vi "Mixed Mode Parameters Popup.vi"(11 "error in (no error)":errorcluster) -> (4 "L1 Param":bool, 6 "L1 Stiff":bool, 8 "L2 Param":bool, 10 "L2 Stiff":bool, 15 "error out":errorcluster)   [LabVIEW 2013]
uses:
  lib/Data Access Objects/Metadata/Cartesian Point.ctl
  lib/Data Access Objects/Metadata/Cartesian Force Vector.ctl
  lib/Data Access Objects/Metadata/Cartesian Force Matrix.ctl
  lib/Data Access Objects/Metadata/Persistant DAO Actions.ctl
  lib/Data Access Objects/Metadata/LBCB Number.ctl
panel:
  in  "Tab Control":enum32{"Parameters", "Stiffness"}(tab)
  in  "Max Increment L1":T1 caption="Max Increment"
  in  "Jacobian Gain L1":T1 caption="Jacobian Gain"
  in  "Force Error Range L1":T2 caption="Force Error Range"
  in  "Max Increment L2":T1 caption="Max Increment"
  in  "Jacobian Gain L2":T1 caption="Jacobian Gain"
  in  "Force Error Range L2":T2 caption="Force Error Range"
  in  "Limit L2 Label 2":string="LBCB 2"
  in  "Jacobian Diagonal LBCB2":dbl[](array[numeric])
  in  "Jacobian Diagonal LBCB1":dbl[](array[numeric])
  in  "Stiffness Limit LBCB2":T3
  in  "Stiffness Limit LBCB1":T3
  in  "Ok":bool
  # "LBCB 1"
  # "dDx"
  # "dDx"
  # "dDy"
  # "dDy"
  # "dDz"
  # "dDz"
  # "dRx"
  # "dRx"
  # "dRy"
  # "dRy"
  # "dRz"
  # "dRz"
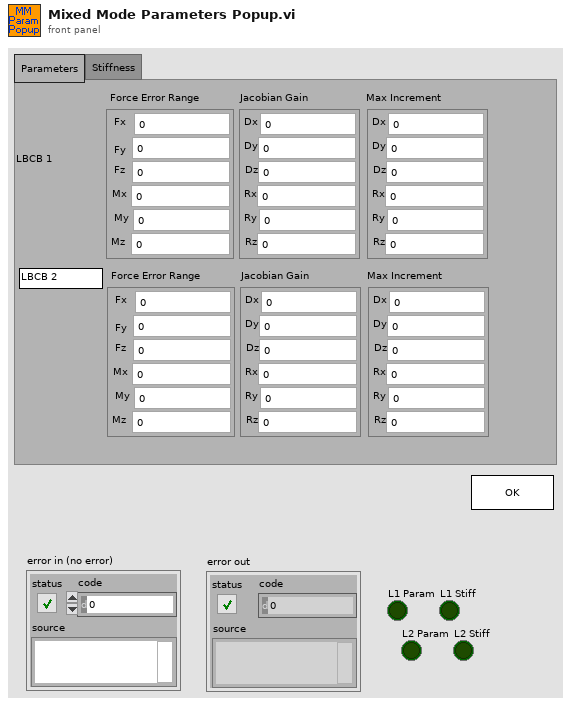
[diagram p1: front panel]
types:
  T1 = typedef "Cartesian Point.ctl" = cluster{"Dx":dbl, "Dy":dbl, "Dz":dbl, "Rx":dbl, "Ry":dbl, "Rz":dbl}
  T2 = typedef "Cartesian Force Vector.ctl" = cluster{"Fx":dbl, "Fy":dbl, "Fz":dbl, "Mx":dbl, "My":dbl, "Mz":dbl}
  T3 = typedef "Cartesian Force Matrix.ctl" = cluster{"Lower":T2, "Upper":T2}
  T4 = typedef "LBCB Number.ctl" = enum16{"LBCB1", "LBCB2"}
  T5 = typedef "Persistant DAO Actions.ctl" = enum16{"Init", "Get", "Set", "Load", "Save"}
  T6 = typedef "Stiffness Matrix.ctl" = dbl[][]
  T7 = typedef "Cartesian Matrix.ctl" = cluster{"Lower":T1, "Upper":T1}
  T8 = typedef "Number Of LBCBs.ctl" = enum16{"1", "2"}
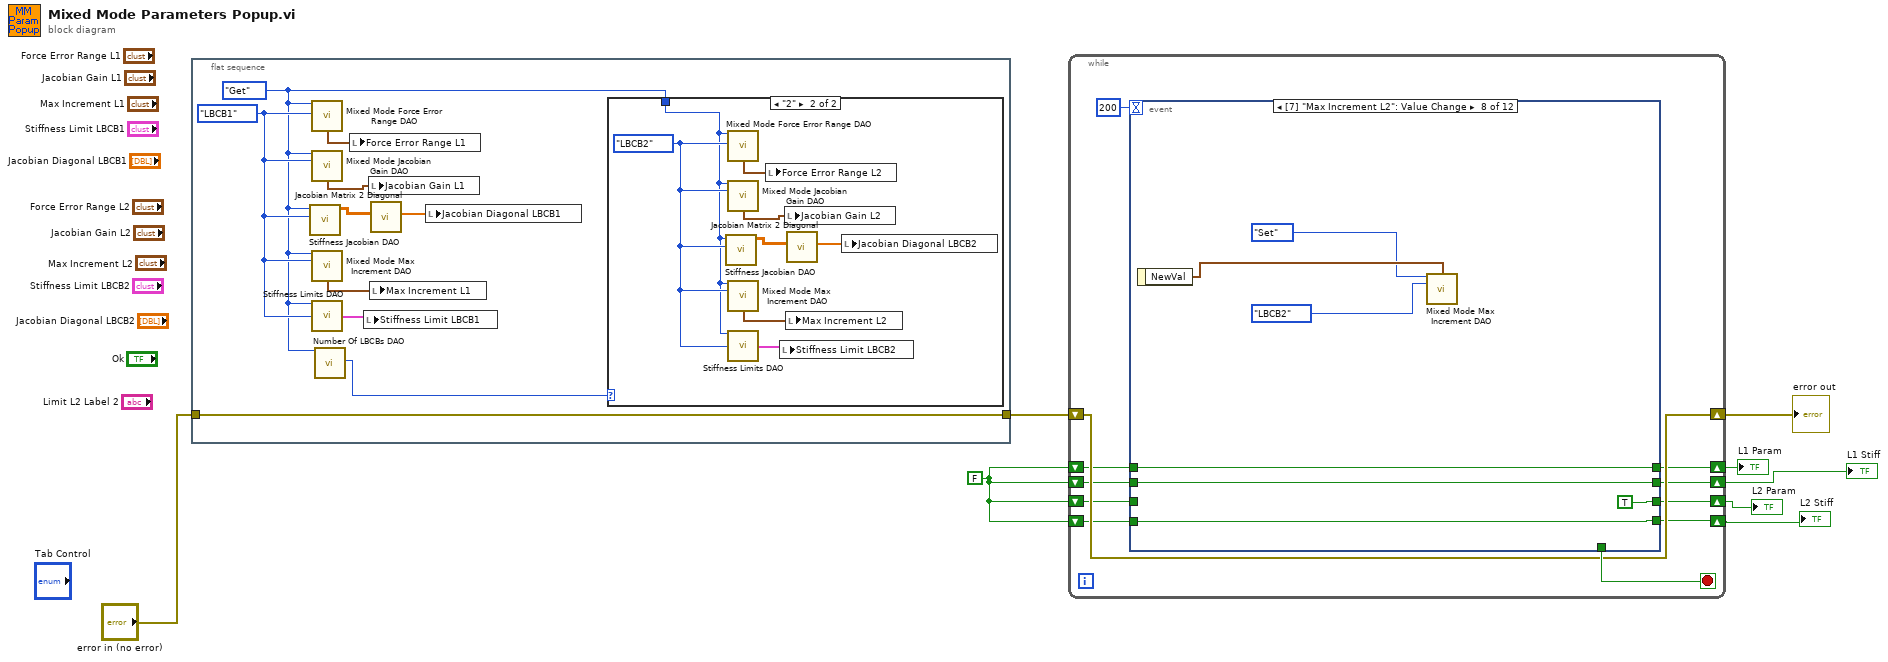
[diagram p0: block diagram]
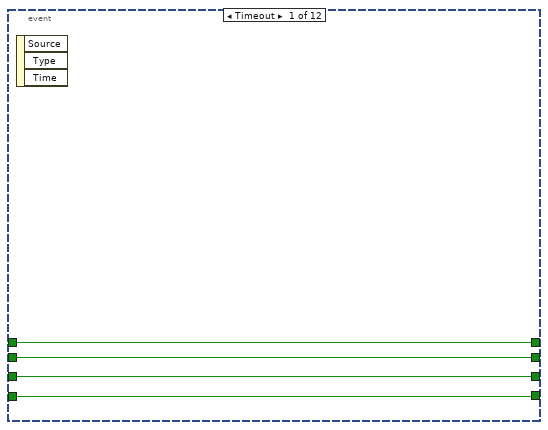
[diagram p2: hidden frame]
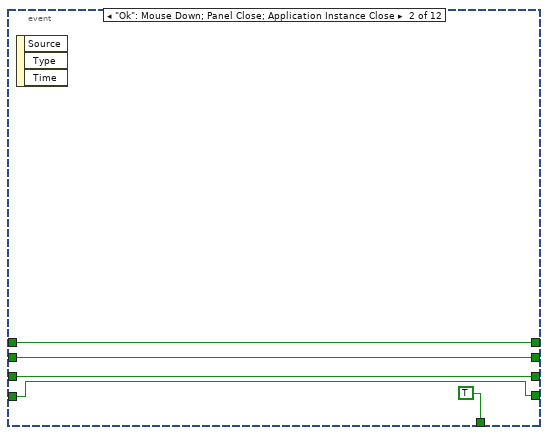
[diagram p3: hidden frame]
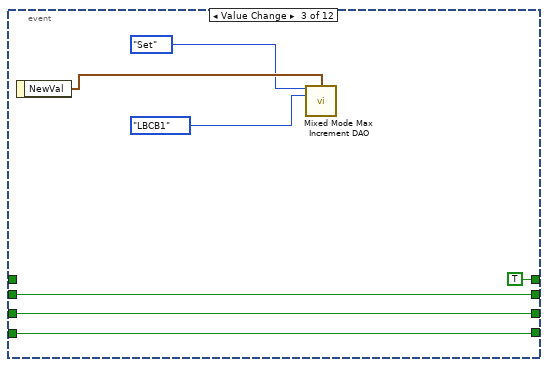
[diagram p4: hidden frame]
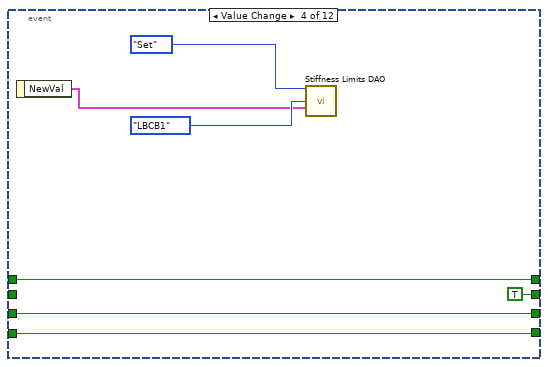
[diagram p5: hidden frame]
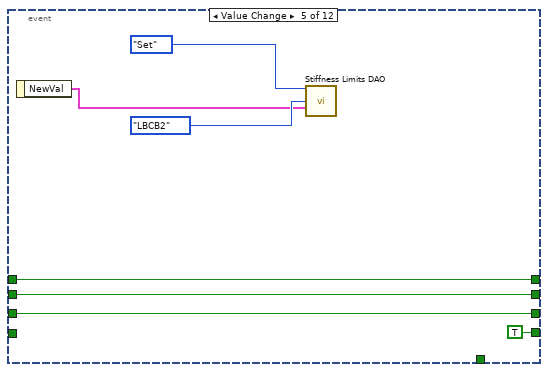
[diagram p6: hidden frame]
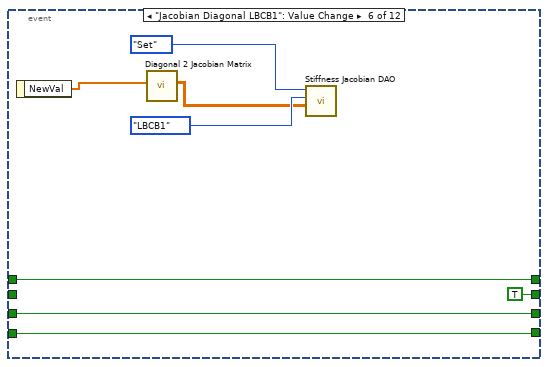
[diagram p7: hidden frame]
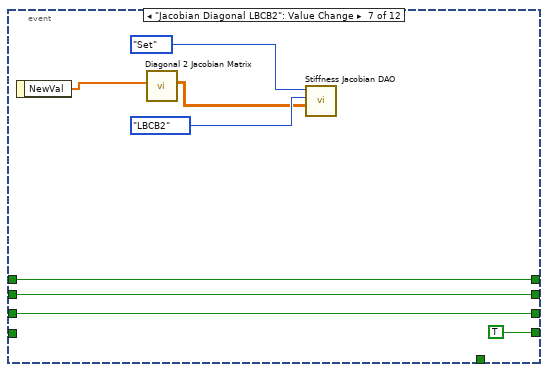
[diagram p8: hidden frame]
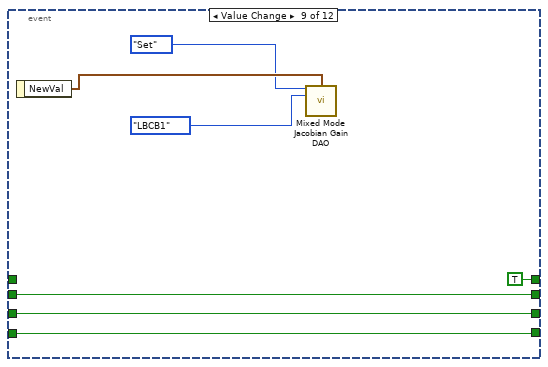
[diagram p9: hidden frame]
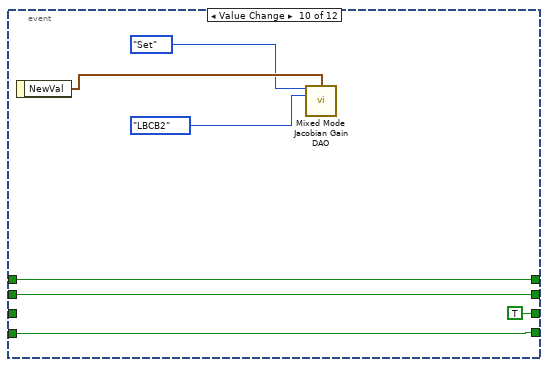
[diagram p10: hidden frame]
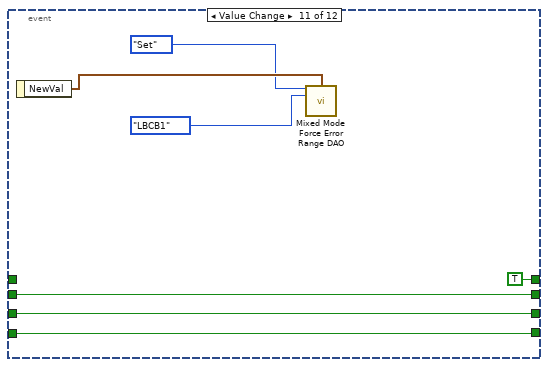
[diagram p11: hidden frame]
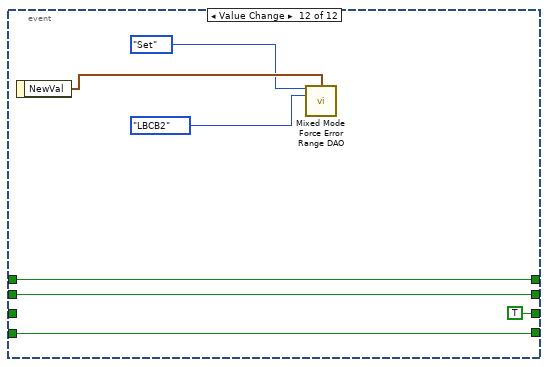
[diagram p12: hidden frame]
diagram:
  w5 = FALSE
  n1 = flat-sequence {
    tunnel: "error in (no error)" -> [w9]
    tunnel: [w9] -> w7
    frame #0 {
      w12 = LBCB_Number."LBCB1" ("LBCB Number")
      w10 = Persistant_DAO_Actions."Get" ("Force Error Range Actions")
      n2 = call "Stiffness Jacobian DAO.vi"("LBCB Number"=w12, "Actions"=w10) -> ("Stiffness Jacobian Out"=w16:T6)  [unwired: 3 in, 6 out]
      n3 = call "Mixed Mode Force Error Range DAO.vi"("Force Error Range Actions"=w10, "LBCB Number"=w12) -> ("Force Error Range Out"=w18:T1)  [unwired: 3 in, 10 out]
      n4 = call "Mixed Mode Jacobian Gain DAO.vi"("Jacobian Gain Actions"=w10, "LBCB Number"=w12) -> ("Jacobian Gain Out"=w17:T1)  [unwired: 3 in, 10 out]
      n5 = call "Mixed Mode Max Increment DAO.vi"("Max Increment Actions"=w10, "LBCB Number"=w12) -> ("Max Increment Out"=w14:T1)  [unwired: 3 in, 10 out]
      n6 = call "Stiffness Limits DAO.vi"("Actions"=w10, "ID"=w12) -> ("Stiffness Limit Out"=w13:T7)  [unwired: 11 in, 2 out]
      n7 = call "Number Of LBCBs DAO.vi"("Actions"=w10) -> ("Number of\nLBCBs Out"=w11:T8)  [unwired: 13 in, 5 out]
      n8 = local write "Force Error Range L1"(w18) -> ()
      n9 = local write "Stiffness Limit LBCB1"(w13) -> ()
      n10 = local write "Jacobian Gain L1"(w17) -> ()
      n11 = local write "Max Increment L1"(w14) -> ()
      n12 = call "Jacobian Matrix 2 Diagonal.vi"("Stiffness Jacobian In"=w16) -> ("Jacobian Diagonal Out"=w15:dbl[])  [unwired: 10 in]
      n13 = local write "Jacobian Diagonal LBCB1"(w15) -> ()
      n14 = case shown="\"2\"" w11 {
        tunnel: w10 -> [_ w19]
        frame "1", Default {
        }
        frame "2" {
          w26 = LBCB_Number."LBCB2" ("LBCB Number")
          n15 = call "Stiffness Jacobian DAO.vi"("LBCB Number"=w26, "Actions"=w19) -> ("Stiffness Jacobian Out"=w22:T6)  [unwired: 3 in, 6 out]
          n16 = call "Mixed Mode Force Error Range DAO.vi"("Force Error Range Actions"=w19, "LBCB Number"=w26) -> ("Force Error Range Out"=w20:T1)  [unwired: 3 in, 10 out]
          n17 = call "Mixed Mode Jacobian Gain DAO.vi"("Jacobian Gain Actions"=w19, "LBCB Number"=w26) -> ("Jacobian Gain Out"=w21:T1)  [unwired: 3 in, 10 out]
          n18 = call "Mixed Mode Max Increment DAO.vi"("Max Increment Actions"=w19, "LBCB Number"=w26) -> ("Max Increment Out"=w24:T1)  [unwired: 3 in, 10 out]
          n19 = call "Stiffness Limits DAO.vi"("Actions"=w19, "ID"=w26) -> ("Stiffness Limit Out"=w25:T7)  [unwired: 11 in, 2 out]
          n20 = local write "Force Error Range L2"(w20) -> ()
          n21 = local write "Stiffness Limit LBCB2"(w25) -> ()
          n22 = local write "Jacobian Gain L2"(w21) -> ()
          n23 = local write "Max Increment L2"(w24) -> ()
          n24 = call "Jacobian Matrix 2 Diagonal.vi"("Stiffness Jacobian In"=w22) -> ("Jacobian Diagonal Out"=w23:dbl[])  [unwired: 10 in]
          n25 = local write "Jacobian Diagonal LBCB2"(w23) -> ()
        }
      }
    }
  }
  n26 = while {
    shift-right: [w35] -> w6
    shift-left: w7 -> [w35]
    shift-right: [w27] -> w4
    shift-left: w5 -> [w30]
    shift-right: [w28] -> w3
    shift-left: w5 -> [w31]
    shift-right: [w29] -> w2
    shift-left: w5 -> [w33]
    shift-right: [w34] -> w1
    shift-left: w5 -> [w32]
    stop <- w36 stop-if-true
    n27 = event shown="[7] \"Max Increment L2\": Value Change" {
      selector: _ -> [_ _ _ _ _ _ _ _ _ _ _ _]
      dyn-events: _ -> [_ _ _ _ _ _ _ _ _ _ _ _]
      timeout: 200 -> [_ _ _ _ _ _ _ _ _ _ _ _]
      tunnel: [_ TRUE _ _ _ _ _ _ _ _ _ _] -> w36
      tunnel: [w38 w42 w47 w54 TRUE w68 TRUE w86 w91 w98 w105 w112] -> w34
      tunnel: w33 -> [w39 w43 w48 w55 w61 w69 w78 _ w92 _ w106 _]
      tunnel: w32 -> [w38 w42 w47 w54 _ w68 _ w86 w91 w98 w105 w112]
      tunnel: w31 -> [w40 w44 w49 _ w62 _ w77 w84 w93 w99 w107 w113]
      tunnel: w30 -> [w41 w45 _ w56 w63 w70 w76 w87 _ w100 _ w114]
      tunnel: [w39 w43 w48 w55 w61 w69 w78 TRUE w92 TRUE w106 TRUE] -> w29
      tunnel: [w40 w44 w49 TRUE w62 TRUE w77 w84 w93 w99 w107 w113] -> w28
      tunnel: [w41 w45 TRUE w56 w63 w70 w76 w87 TRUE w100 TRUE w114] -> w27
      event Timeout {
        n28 = event-data() -> ()  [unwired: 1 in, 3 out]
      }
      event "Ok": Mouse Down; Panel Close; Application Instance Close {
        n29 = event-data() -> ()  [unwired: 1 in, 3 out]
      }
      event Value Change {
        n30 = event-data() -> ("NewVal"=w53:T1)  [unwired: 1 in]
        n31 = call "Mixed Mode Max Increment DAO.vi"("Max Increment Actions"=Persistant_DAO_Actions."Set", "Max Increment In"=w53, "LBCB Number"=LBCB_Number."LBCB1") -> ()  [unwired: 2 in, 11 out]
      }
      event Value Change {
        n32 = event-data() -> ("NewVal"=w58:T3)  [unwired: 1 in]
        n33 = call "Stiffness Limits DAO.vi"("Actions"=Persistant_DAO_Actions."Set" ("Max Increment Actions"), "ID"=LBCB_Number."LBCB1" ("LBCB Number"), "Stiffness Limit In"=w58) -> ()  [unwired: 10 in, 3 out]
      }
      event Value Change {
        n34 = event-data() -> ("NewVal"=w65:T3)  [unwired: 1 in]
        n35 = call "Stiffness Limits DAO.vi"("Actions"=Persistant_DAO_Actions."Set" ("Max Increment Actions"), "ID"=LBCB_Number."LBCB2" ("LBCB Number"), "Stiffness Limit In"=w65) -> ()  [unwired: 10 in, 3 out]
      }
      event "Jacobian Diagonal LBCB1": Value Change {
        n36 = event-data() -> ("NewVal"=w73:dbl[])  [unwired: 1 in]
        n37 = call "Diagonal 2 Jacobian Matrix.vi"("Jacobian Diagonal Out"=w73) -> ("Stiffness Jacobian In"=w72:T6)  [unwired: 10 in]
        n38 = call "Stiffness Jacobian DAO.vi"("Stiffness Jacobian In"=w72, "LBCB Number"=LBCB_Number."LBCB1", "Actions"=Persistant_DAO_Actions."Set" ("Max Increment Actions")) -> ()  [unwired: 6 in, 3 out]
      }
      event "Jacobian Diagonal LBCB2": Value Change {
        n39 = event-data() -> ("NewVal"=w81:dbl[])  [unwired: 1 in]
        n40 = call "Diagonal 2 Jacobian Matrix.vi"("Jacobian Diagonal Out"=w81) -> ("Stiffness Jacobian In"=w80:T6)  [unwired: 10 in]
        n41 = call "Stiffness Jacobian DAO.vi"("Stiffness Jacobian In"=w80, "LBCB Number"=LBCB_Number."LBCB2", "Actions"=Persistant_DAO_Actions."Set" ("Max Increment Actions")) -> ()  [unwired: 6 in, 3 out]
      }
      event Value Change {
        n42 = event-data() -> ("NewVal"=w90:T1)  [unwired: 1 in]
        n43 = call "Mixed Mode Max Increment DAO.vi"("Max Increment Actions"=Persistant_DAO_Actions."Set", "Max Increment In"=w90, "LBCB Number"=LBCB_Number."LBCB2") -> ()  [unwired: 2 in, 11 out]
      }
      event Value Change {
        n44 = event-data() -> ("NewVal"=w97:T1)  [unwired: 1 in]
        n45 = call "Mixed Mode Jacobian Gain DAO.vi"("Jacobian Gain Actions"=Persistant_DAO_Actions."Set" ("Max Increment Actions"), "Jacobian Gain In"=w97, "LBCB Number"=LBCB_Number."LBCB1") -> ()  [unwired: 10 in, 3 out]
      }
      event Value Change {
        n46 = event-data() -> ("NewVal"=w104:T1)  [unwired: 1 in]
        n47 = call "Mixed Mode Jacobian Gain DAO.vi"("Jacobian Gain Actions"=Persistant_DAO_Actions."Set" ("Max Increment Actions"), "Jacobian Gain In"=w104, "LBCB Number"=LBCB_Number."LBCB2") -> ()  [unwired: 10 in, 3 out]
      }
      event Value Change {
        n48 = event-data() -> ("NewVal"=w111:T2)  [unwired: 1 in]
        n49 = call "Mixed Mode Force Error Range DAO.vi"("Force Error Range Actions"=Persistant_DAO_Actions."Set" ("Max Increment Actions"), "Force Error Range In"=w111, "LBCB Number"=LBCB_Number."LBCB1") -> ()  [unwired: 10 in, 3 out]
      }
      event Value Change {
        n50 = event-data() -> ("NewVal"=w118:T2)  [unwired: 1 in]
        n51 = call "Mixed Mode Force Error Range DAO.vi"("Force Error Range Actions"=Persistant_DAO_Actions."Set" ("Max Increment Actions"), "Force Error Range In"=w118, "LBCB Number"=LBCB_Number."LBCB2") -> ()  [unwired: 10 in, 3 out]
      }
    }
  }
  "error out" <- w6
  "L1 Param" <- w4
  "L1 Stiff" <- w3
  "L2 Param" <- w2
  "L2 Stiff" <- w1
